vi "dependency-callerregistration-test.vi"(8 "error in (no error)":errorcluster) -> (0 "error out":errorcluster)   [LabVIEW 2013]
uses:
  _test-support-SMOs/SMO.Configurable/Config--cluster.ctl
  _test-support-SMOs/SMO.Configurable/SMO.Configurable.lvclass
  src/SMO/SMO.lvclass
  <vilib>/addons/_JKI Toolkits/Caraya/classes/Test/Test.lvclass
  <vilib>/addons/_JKI Toolkits/Caraya/classes/Assert/Assert.lvclass
panel:
  out "Dependency Config event received":bool
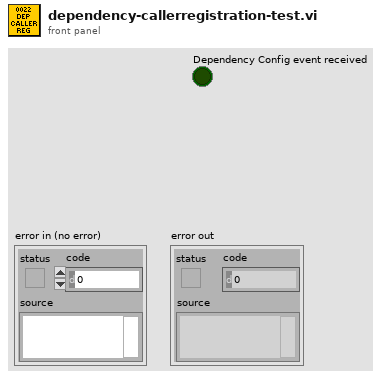
[diagram p1: front panel]
types:
  T1 = typedef "SMO.Configurable.lvclass/Config--cluster.ctl" = cluster{"timeout":i32, "run":bool}
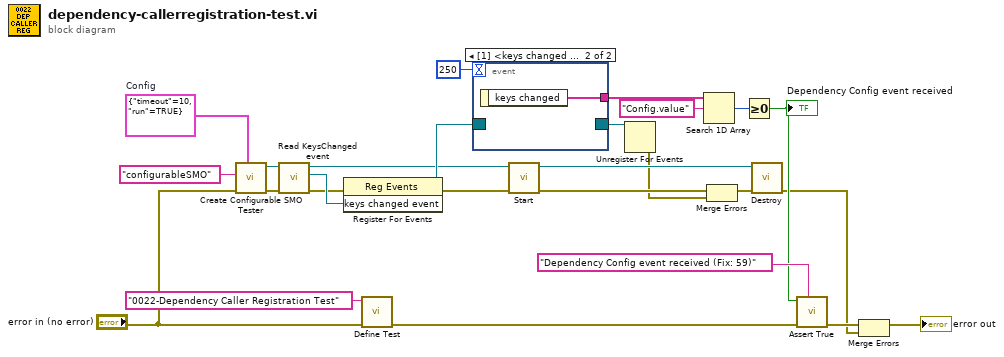
[diagram p0: block diagram]
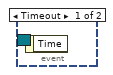
[diagram p2: hidden frame]
diagram:
  w25 = T1 {"timeout"=10, "run"=TRUE}  # Config
  n1 = call "Create Configurable SMO Tester.vi"("Config"=w25, "error in (no error)"="error in (no error)", "Subsystem Name (optional)"="configurableSMO") -> ("error out"=w16:errorcluster, "SMO.Configurable out"=w17:refnum<class "SMO.Configurable.lvclass">)  [unwired: 6 in, 1 out]
  n2 = call "Read KeysChanged event.vi"("error in (no error)"=w16, "SMO.Configurable in"=w17) -> ("error out"=w13:errorcluster, "keys changed event"=w15:refnum<user-event>, "SMO.Configurable out"=w14:refnum<class "SMO.Configurable.lvclass">)  [unwired: 7 in]
  n3 = register-events(error in=w13, w15) -> (reference out=w20:refnum<event-registration>, error out=w21:errorcluster)  [unwired: 1 in]
  n4 = call <vilib>:"Define Test.vi"("error in (no error)"="error in (no error)", "Label (VI Title)"="0022-Dependency Caller Registration Test") -> ("error out"=w6:errorcluster)  [unwired: 9 in]
  n5 = event shown="[1] <keys changed event>: User Event" {
    selector: w20 -> [_ _]
    dyn-events: [_ _] -> w19
    timeout: 250 -> [_ _]
    tunnel: [_ w27] -> w11
    event Timeout {
      n6 = event-data() -> ()  [unwired: 1 in, 1 out]
    }
    event User Event {
      n7 = event-data() -> ("keys changed"=w27:string[])  [unwired: 1 in]
    }
  }
  n8 = call "Start.vi"("error in (no error)"=w21, "SMO"=w14) -> ("error out"=w22:errorcluster, "SMO out"=w24:refnum<class "SMO.Configurable.lvclass">)  [unwired: 8 in]
  n9 = Unregister For Events(event registration refnum=w19) -> (error out=w18:errorcluster)  [unwired: 1 in]
  n10 = Search 1D Array(1D array=w11, element="Config.value") -> (index of element=w9:i32)  [unwired: 1 in]
  n11 = Merge Errors(w22, w18) -> (w23:errorcluster)
  n12 = Greater Or Equal To 0?(x=w9) -> (x >= 0?=w7:bool)
  "Dependency Config event received" <- w7
  n13 = call "Destroy.vi"("error in (no error)"=w23, "SMO"=w24) -> ("error out"=w3:errorcluster)  [unwired: 9 in]
  n14 = call <vilib>:"Assert True.vi"("Label"="Dependency Config event received (Fix: 59)", "error in (no error)"=w6, "True?"=w7) -> ("error out"=w5:errorcluster)  [unwired: 8 in]
  n15 = Merge Errors(w5, w3) -> (→"error out":errorcluster)
